vi "Magnet fit.vi"(1 "Coefficients":dbl[](array[numeric])=[0.0, 1.0, 0.0] format="%.5e", 2 "Magnet Parameter":dbl=1.0 format="%.4f") -> (0 "Conjugate Parameter":dbl=1.0 format="%.4f")   [LabVIEW 2020]
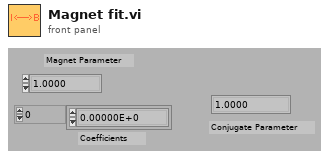
[diagram p1: front panel]
types:
  T1 = cluster{"Coefficients[0]":dbl, "Coefficients[1]":dbl, "Coefficients[2]":dbl}
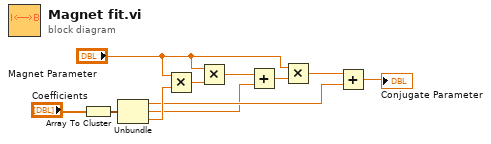
[diagram p0: block diagram]
diagram:
  n1 = Array To Cluster(array="Coefficients") -> (cluster=w7:T1)
  n2 = Unbundle(w7) -> ("Coefficients[0]"=w5:dbl, "Coefficients[1]"=w2:dbl, "Coefficients[2]"=w6:dbl)
  n3 = Multiply(x="Magnet Parameter", y=w6) -> (x*y=w10:dbl)
  n4 = Multiply(x="Magnet Parameter", y=w10) -> (x*y=w3:dbl)
  n5 = Add(x=w3, y=w2) -> (x+y=w4:dbl)
  n6 = Multiply(x="Magnet Parameter", y=w4) -> (x*y=w9:dbl)
  n7 = Add(x=w9, y=w5) -> (x+y=→"Conjugate Parameter":dbl)
